vi "OAT STFT Spectrogram at Indices (Continuous).vi"(0 "resampled signal":waveform(dbl)={"t0"=timestamp(0 s since 1904-01-01), "dt"=0.0, "Y"=[]}, 1 "dB On (T)":bool=TRUE, 3 "reset? (True)":bool=TRUE, 5 "time indices":dbl[](array[numeric]) format="%.2f", 7 "X scale in":cluster{"offset":dbl, "multiplier":dbl} {"multiplier" format="%.2f"; "offset" format="%.2f"}, 9 "last indices":dbl format="%.2f", 11 "error in (no error)":errorcluster, 12 "spectral settings":T2={"window type"=1, "number of lines"=400} {"number of lines" min=2; "window type" items=["None"=0, "Hanning"=1, "Hamming"=2, "Blackman-Harris"=3, "Exact Blackman"=4, "Blackman"=5, "Flat Top"=6, "4 Term B-Harris"=7, "7 Term B-Harris"=8, "Low Sidelobe"=9, "Gaussian"=62]}) -> (4 "spectral map":dbl[][](array[numeric]) format="%.2f", 6 "scales":T1 {"Y scale"."multiplier" format="%.2f"; "Y scale"."offset" format="%.2f"; "X scale"."multiplier" format="%.2f"; "X scale"."offset" format="%.2f"}, 10 "Z axis unit label":string, 14 "finished":bool, 15 "error out":errorcluster)   [LabVIEW 2017, in "SoundVib_Resampling.lvlib"]
doc: "Computes Short Time Fourier Transform spectrogram at specified indices."
uses:
  <vilib>/addons/Sound and Vibration/Order Analysis/Resample Order Tracking/SoundVib_Resampling.lvlib
  <vilib>/addons/_NISVFA/_Shared subVIs/Common/svc_Engineering Units to Unit Label.vi
  <vilib>/addons/_NISVFA/_Shared subVIs/Common/svc_Unit Label to Engineering Units.vi
  <vilib>/Analysis/NI_AALPro.lvlib
panel:
  # "STFT Spectrogram at Indices"
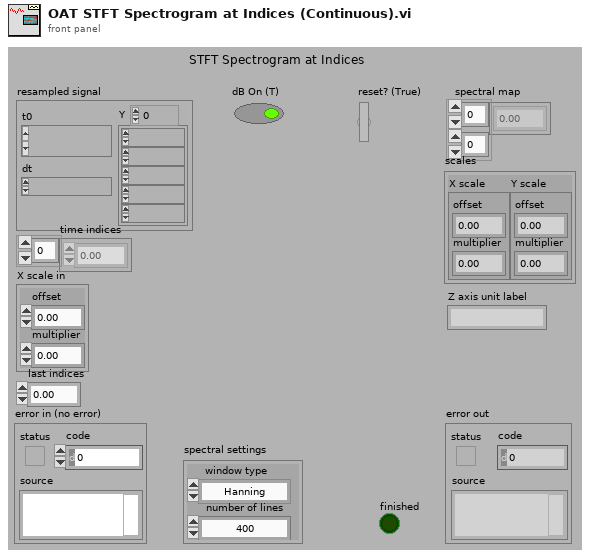
[diagram p1: front panel]
types:
  T1 = cluster{"X scale":cluster{"offset":dbl, "multiplier":dbl}, "Y scale":cluster{"offset":dbl, "multiplier":dbl}}
  T2 = cluster{"window type":u32, "number of lines":i32}
  T3 = typedef "svc_Channel Info.ctl" = cluster{"sensor sensitivity":dbl, "engineering units":T4, "dB reference":dbl, "custom label":string, "weighting filter":T5, "pregain":dbl}
  T4 = typedef "svc_Engineering Units Text Ring.ctl" = u16
  T5 = typedef "svc_Weighting Filter Text Ring.ctl" = u16
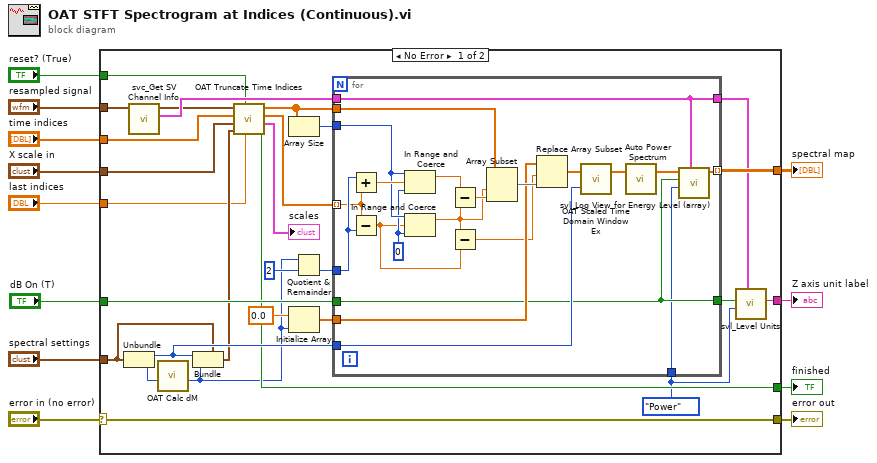
[diagram p0: block diagram]
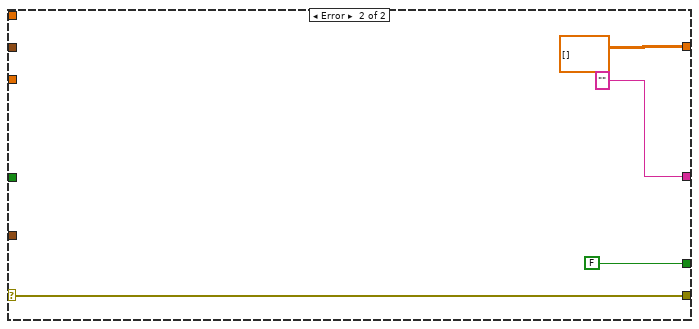
[diagram p2: hidden frame]
diagram:
  n1 = case shown="No Error" "error in (no error)" {
    selector: "error in (no error)" -> [w17 w65]
    tunnel: "dB On (T)" -> [w35 _]
    tunnel: [w34 dbl[][] [] ("log view [dB EU]")] -> w11
    tunnel: "time indices" -> [w32 _]
    tunnel: "resampled signal" -> [w30 _]
    tunnel: "spectral settings" -> [w27 _]
    tunnel: "reset? (True)" -> [w26 _]
    tunnel: [w23 FALSE ("finished")] -> w6
    tunnel: "X scale in" -> [w22 _]
    tunnel: "last indices" -> [w18 _]
    tunnel: [w17 w65] -> w2
    tunnel: [w13 "" ("unit label")] -> w1
    frame No Error {
      w14 = enum16{"Power", "Amplitude"}."Power" ("view mode")
      n2 = Unbundle(w27) -> ("window type"=w28:u32, "number of lines"=w29:i32)
      n3 = call <vilib>:"svc_Get SV Channel Info.vi"("scaled signal [EU]"=w30) -> ("channel info"=w33:T3, "dup scaled signal [EU]"=w25:waveform(dbl))  [unwired: 5 in, 4 out]
      n4 = call <vilib>:"OAT Calc dM.vi"("window length"=w29) -> ("actual window length"=w20:i32)  [unwired: 7 in, 3 out]
      n5 = Bundle(cluster=w27, "window type"=w28, "number of lines"=w20) -> (w21:T2)
      n6 = call <vilib>:"OAT Truncate Time Indices.vi"("last indices"=w18, "reset? (True)"=w26, "spectral settings"=w21, "X scale in"=w22, "time in"=w32, "scaled signal [EU] in"=w25) -> ("finished"=w23:bool, "scales"=→"scales":T1, "window indices"=w24:dbl[], "data out"=w31:dbl[])  [unwired: 2 in]
      n7 = Array Size(array=w31) -> (size(s)=w38:i32)
      n8 = Initialize Array(0.0 ("Element Data"), w20) -> (w36:dbl[])
      n9 = Quotient & Remainder(x=w20, y=2) -> (floor(x/y)=w39:i32)  [unwired: 1 out]
      n10 = for {
        tunnel: w31 -> [w52]
        tunnel: w24 -> [w60] mode=indexing
        tunnel: w39 -> [w61]
        tunnel: w38 -> [w58]
        tunnel: w36 -> [w50]
        tunnel: [w44] -> w34 mode=indexing
        tunnel: w28 -> [w46]
        tunnel: w35 -> [w42]
        tunnel: w33 -> [w43]
        tunnel: [w43] -> w16
        tunnel: [w42] -> w15
        tunnel: w14 -> [w41]
        w57 = 0 ("lower limit")
        n11 = Add(x=w61, y=w60) -> (x+y=w59:dbl)
        n12 = Subtract(x=w60, y=w61) -> (x-y=w55:dbl)
        n13 = In Range and Coerce(upper limit=w58, x=w59, lower limit=w57) -> (coerced(x)=w56:dbl)  [unwired: 1 out]
        n14 = In Range and Coerce(upper limit=w58, x=w55, lower limit=w57) -> (coerced(x)=w53:dbl)  [unwired: 1 out]
        n15 = Subtract(x=w56, y=w53) -> (x-y=w54:dbl)
        n16 = Subtract(x=w53, y=w55) -> (x-y=w49:dbl)
        n17 = Array Subset(array=w52, index=w53, length=w54) -> (w51:dbl[])
        n18 = Replace Array Subset(array=w50, new element=w51, index=w49) -> (w48:dbl[])
        n19 = call <vilib>:"OAT Scaled Time Domain Window Ex.vi"("window type"=w46, "X"=w48) -> ("y"=w47:dbl[])  [unwired: 1 out]
        n20 = call <vilib>:"Auto Power Spectrum.vi"("Signal (V)"=w47) -> ("Power Spectrum (V^2 rms)"=w45:dbl[])  [unwired: 1 in, 1 out]
        n21 = call <vilib>:"svl_Log View for Energy Level (array).vi"("channel info"=w43, "view mode"=w41, "dB On (T)"=w42, "scaled signal"=w45) -> ("log view scaled signal"=w44:dbl[])  [unwired: 5 in, 2 out]
      }
      n22 = call <vilib>:"svl_Level Units.vi"("channel info"=w16, "view mode"=w14, "dB On (T)"=w15) -> ("unit label"=w13:string)  [unwired: 6 in, 2 out]
    }
    frame Error {
    }
  }
  "spectral map" <- w11
  "Z axis unit label" <- w1
  "finished" <- w6
  "error out" <- w2
